vi "Step2.vi"() -> ()   [LabVIEW 2025]
uses:
  <vilib>/Utility/file.llb/Read Delimited Spreadsheet (DBL).vi
  <vilib>/Analysis/NI_AALBase.lvlib
panel:
  out "Waveform Graph":dynamicdata(graph)
  out "After Outlier Removal":waveform(dbl)(graph)
  in  "Z Threshold":dbl
  in  "Data File Path":path
  out "Time vs Signal":waveform(dbl)(graph)
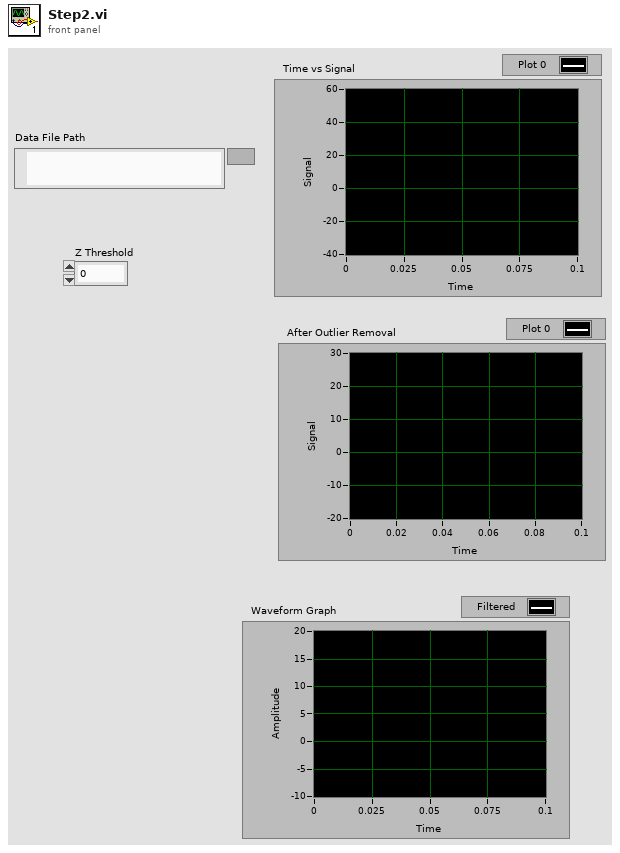
[diagram p1: front panel]
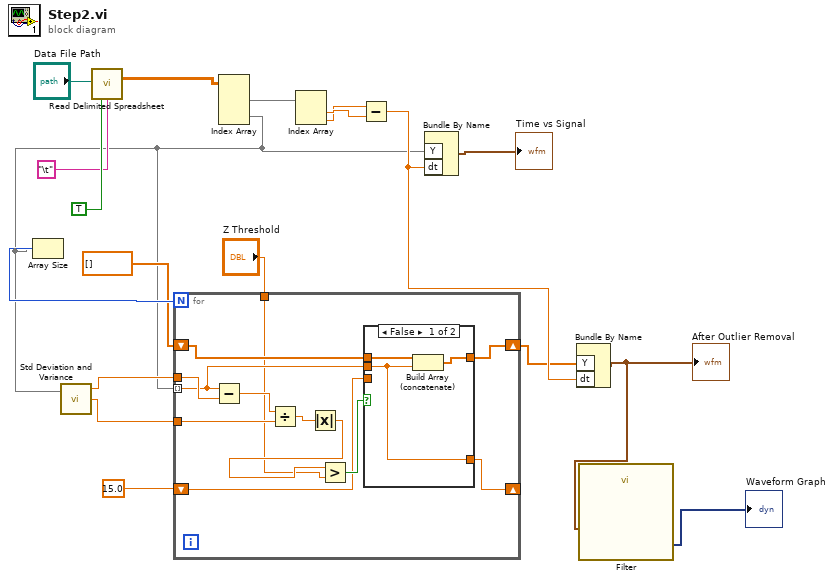
[diagram p0: block diagram]
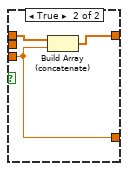
[diagram p2: hidden frame]
diagram:
  n1 = call-poly <vilib>:"Read Delimited Spreadsheet.vi"("file path (dialog if empty)"="Data File Path", "transpose? (F)"=TRUE, "delimiter (\\t)"="\t" ("delimiter (\\t)")) -> ("all rows"=w17:dbl[][])  [unwired: 7 in, 5 out]
  n2 = Index Array(array=w17) -> (element #1=w16:dbl[], element #2=w3:dbl[])  [unwired: 4 in]
  n3 = Array Size(array=w3) -> (size(s)=w11:i32)
  n4 = call <vilib>:"Std Deviation and Variance.vi"("X"=w3) -> ("mean"=w10:dbl, "standard deviation"=w9:dbl)  [unwired: 1 in, 1 out]
  n5 = for {
    N: w11 -> [_]
    shift-right: [w26] -> w5
    tunnel: w9 -> [w30]
    tunnel: w3 -> [w24] mode=indexing
    tunnel: w10 -> [w28]
    tunnel: "Z Threshold" -> [w20]
    shift-left: dbl[] [] -> [w25]
    shift-right: [w22] -> _
    shift-left: 15.0 -> [w23]
    n6 = Subtract(x=w24, y=w28) -> (x-y=w31:dbl)
    n7 = Divide(x=w31, y=w30) -> (x/y=w29:dbl)
    n8 = Absolute Value(x=w29) -> (abs(x)=w21:dbl)
    n9 = Greater?(x=w21, y=w20) -> (0:w27:bool)
    n10 = case shown="False" w27 {
      tunnel: w24 -> [w32 _]
      tunnel: w25 -> [w33 w37]
      tunnel: [w34 w36] -> w26
      tunnel: w23 -> [_ w35]
      tunnel: [w32 w35] -> w22
      frame False {
        n11 = Build Array (concatenate)(w33, w32) -> (w34:dbl[])
      }
      frame True {
        n12 = Build Array (concatenate)(w37, w35) -> (w36:dbl[])
      }
    }
  }
  n13 = Index Array(array=w16) -> (element #1=w15:dbl, element #2=w4:dbl)  [unwired: 2 in]
  n14 = Subtract(x=w4, y=w15) -> (x-y=w6:dbl)
  n15 = Bundle By Name("Y"=w3, "dt"=w6) -> (→"Time vs Signal":waveform(dbl))  [unwired: 1 in]
  n16 = Bundle By Name("Y"=w5, "dt"=w6) -> (w1:waveform(dbl))  [unwired: 1 in]
  "After Outlier Removal" <- w1
  n17 = call "Filter"("Signal"=w1) -> ("Filtered Signal"=→"Waveform Graph":dynamicdata)  [unwired: 9 in, 1 out]
